vi "FileIntialize.vi"(8 "Error In":errorcluster, 9 "Labels":string[](array[string]), 11 "refnum in":refnum<file>) -> (0 "Error Out":errorcluster, 3 "File Refnum":refnum<file>)   [LabVIEW 2020]
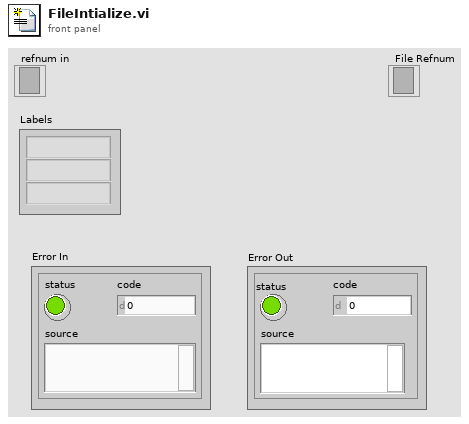
[diagram p1: front panel]
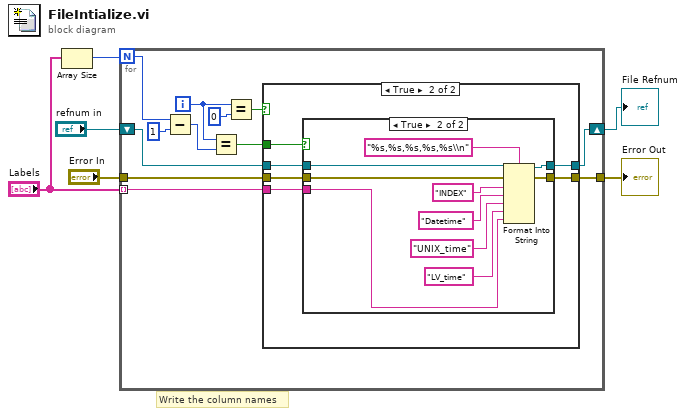
[diagram p0: block diagram]
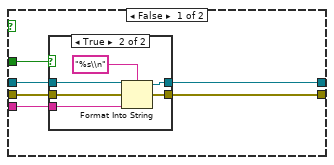
[diagram p2: hidden frame]
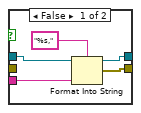
[diagram p3: hidden frame]
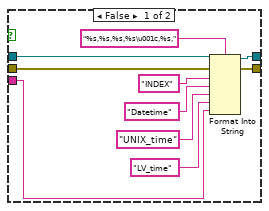
[diagram p4: hidden frame]
diagram:
  # "Write the column names"
  n1 = Array Size(array="Labels") -> (size(s)=w5:i32)
  n2 = for {
    N: w5 -> [w10]
    tunnel: [w13] -> w4
    tunnel: "Labels" -> [w12] mode=indexing
    tunnel: "Error In" -> [w11]
    shift-right: [w7] -> w1
    shift-left: "refnum in" -> [w18]
    i -> [w15]
    n3 = Subtract(x=w10, y=1 ("x")) -> (x-y=w9:i32)
    n4 = Equal?(x=w15, y=w9) -> (x = y?=w14:bool)
    n5 = Equal?(x=w15, y=0) -> (x = y?=w16:bool)
    n6 = case shown="True" w16 {
      tunnel: w18 -> [w24 w41]
      tunnel: w14 -> [w23 w40]
      tunnel: [w22 w38] -> w13
      tunnel: [w21 w39] -> w7
      tunnel: w12 -> [w20 w37]
      tunnel: w11 -> [w19 w36]
      frame False {
        n7 = case shown="True" w23 {
          tunnel: w24 -> [w28 w35]
          tunnel: [w27 w33] -> w22
          tunnel: [w26 w32] -> w21
          tunnel: w20 -> [w25 w31]
          tunnel: w19 -> [_ w30]
          frame False {
            n8 = Format Into String(format string="%s,", initial string=w28, w25) -> (resulting string=w26:refnum<file>, error out=w27:errorcluster)  [unwired: 1 in]
          }
          frame True {
            n9 = Format Into String(format string="%s\\n", initial string=w35, error in=w30, w31) -> (resulting string=w32:refnum<file>, error out=w33:errorcluster)
          }
        }
      }
      frame True {
        n10 = case shown="True" w40 {
          tunnel: w41 -> [w46 w61]
          tunnel: [w44 w55] -> w39
          tunnel: [w45 w54] -> w38
          tunnel: w37 -> [w43 w53]
          tunnel: w36 -> [w42 w52]
          frame False {
            n11 = Format Into String(format string="%s,%s,%s,%s\u001c,%s,", initial string=w46, error in=w42, "INDEX" ("input 1"), "Datetime" ("input 1"), "UNIX_time" ("input 1"), "LV_time" ("input 1"), w43) -> (resulting string=w44:refnum<file>, error out=w45:errorcluster)
          }
          frame True {
            n12 = Format Into String(format string="%s,%s,%s,%s,%s\\n", initial string=w61, error in=w52, "INDEX" ("input 1"), "Datetime" ("input 1"), "UNIX_time" ("input 1"), "LV_time" ("input 1"), w53) -> (resulting string=w55:refnum<file>, error out=w54:errorcluster)
          }
        }
      }
    }
  }
  "File Refnum" <- w1
  "Error Out" <- w4
